vi "Handle Last Ack Core.vi"(4 "error in (no error)":errorcluster, 6 "Last Ack":refnum<class "Last Ack.lvclass">, 7 "MultiplexedConnectionHandler in":refnum<class "MultiplexedConnectionHandler.lvclass">) -> (0 "error out":errorcluster, 3 "MultiplexedConnectionHandler out":refnum<class "MultiplexedConnectionHandler.lvclass">)   [LabVIEW 2019, in "MultiplexedConnectionHandler.lvlib" / "MultiplexedConnectionHandler.lvclass"]
doc: "(<B>Filename</B>: Actor Framework.lvlib:Actor.lvclass:Handle Last Ack Core.vi)\n\nDefines how the caller actor responds to the Last Ack message from a nested actor. The Last Ack message is the final message a nested actor sends to its caller before it shuts down. The message contains information about the final state of the nested actor.\n\nBy default, this method does nothing except return any error the nested actor sent. A descendant class may override this method to define behavior."
uses:
  <vilib>/gpm_packages/@cs/Network-interface/Source/MultiplexedConnectionHandler/MultiplexedConnectionHandler/MultiplexedConnectionHandler.lvclass
  <vilib>/ActorFramework/LastAck/Last Ack.lvclass
  C:/Program Files/National Instruments/LabVIEW 2019/vi.lib/gpm_packages/@cs/Network-interface/Source/PersistantConnectionHandler/PersistantConnectionHandler/PersistantConnectionHandler.lvclass
  C:/Program Files/National Instruments/LabVIEW 2019/vi.lib/gpm_packages/@cs/Network-interface/Source/Logged Actor/LoggedActor.lvclass
  <vilib>/gpm_packages/@cs/Network-interface/Source/ConnectionManager/ConnectionManager/ConnectionManager.lvclass
  <vilib>/gpm_packages/@cs/event-logger/Source/Composed Log/Types/Log Level.ctl
  <vilib>/ActorFramework/LastAck/Last Ack.lvclass/Last Ack.ctl
  <vilib>/gpm_packages/@cs/Network-interface/Source/PersistantConnectionHandler/PersistantConnectionHandler/PersistantConnectionHandler.lvclass/PersistantConnectionHandler.ctl
  <vilib>/gpm_packages/@cs/Network-interface/Source/MultiplexedConnectionHandler/MultiplexedConnectionHandler/MultiplexedConnectionHandler.lvclass/MultiplexedConnectionHandler.ctl
  <vilib>/gpm_packages/@cs/Network-interface/Source/ConnectionManager/ConnectionManager/ConnectionManager.lvclass/ConnectionManager.ctl
  <vilib>/ActorFramework/Message Enqueuer/Message Enqueuer.lvclass
  <vilib>/gpm_packages/@cs/Network-interface/Source/Connection Reference/Connection Reference/Connection Reference.lvclass
  <vilib>/gpm_packages/@cs/Network-interface/Source/Logged Actor/LoggedActor.lvclass/LoggedActor.ctl
  <vilib>/gpm_packages/@cs/event-logger/Source/Composed Log/LoggerReference/LoggerReference.lvclass/LoggerReference.ctl
  <vilib>/gpm_packages/@cs/event-logger/Source/Composed Log/LoggerReference/Log Event.vi
  <vilib>/gpm_packages/@cs/event-logger/Source/Composed Log/LoggerReference/Log.vi
  <vilib>/gpm_packages/@cs/event-logger/Source/Composed Log/LoggerReference/Get Valid Event Time.vi
  <vilib>/gpm_packages/@cs/event-logger/Source/Composed Log/LoggerReference/Remove Stale Logs.vi
  <vilib>/gpm_packages/@cs/Network-interface/Source/MessagingInterfaces/IConnectionStateChangeCallback/IConnectionStateChangeCallback.lvclass
  <vilib>/gpm_packages/@cs/Network-interface/Source/Logged Actor/LoggedActor.lvclass
  <vilib>/gpm_packages/@cs/event-logger/Source/Composed Log/Composed Log.lvlib
  <vilib>/gpm_packages/@cs/Network-interface/Source/PersistantConnectionHandler/PersistantConnectionHandler/PersistantConnectionHandler.lvclass
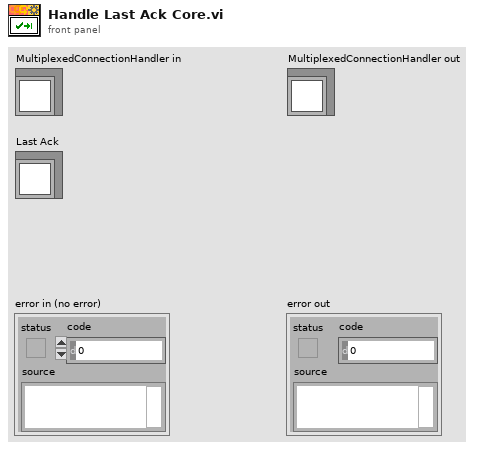
[diagram p1: front panel]
types:
  T1 = typedef "Composed Log.lvlib/Log Level.ctl" = enum16{"Debug", "Info", "Warning", "Error", "Critical"}
  T2 = cluster{"Connection Manager Queue":refnum<class "Message Enqueuer.lvclass">, "Connection Reference":refnum<data-value>}
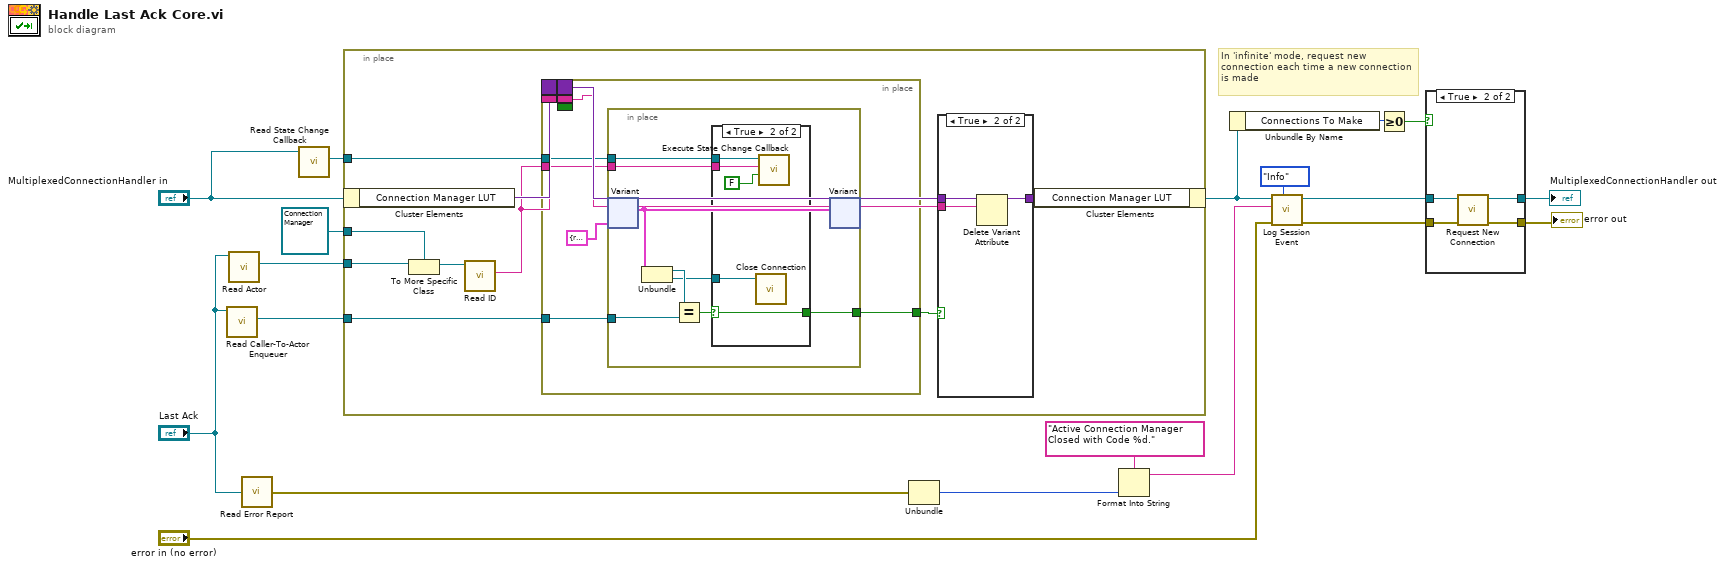
[diagram p0: block diagram]
diagram:
  # "In 'infinite' mode, request new connection each time a new connection is made"
  n1 = call <vilib>:"Read Caller-To-Actor Enqueuer.vi"("Last Ack"="Last Ack") -> ("Caller-to-Actor Enqueuer"=w15:refnum<class "Message Enqueuer.lvclass">)  [unwired: 10 in]
  n2 = call <vilib>:"Read Actor.vi"("Last Ack"="Last Ack") -> ("Actor"=w11:refnum<class "Actor.lvclass">)  [unwired: 10 in]
  n3 = call <vilib>:"Read Error Report.vi"("Last Ack"="Last Ack") -> ("error report"=w19:errorcluster)
  n4 = call <vilib>:"Read State Change Callback.vi"("PersistantConnectionHandler in"="MultiplexedConnectionHandler in") -> ("State Change Callback"=w1:refnum<class "IConnectionStateChangeCallback.lvclass">)  [unwired: 9 in, 1 out]
  n5 = in-place {
    in-place-border: w15 -> [w29]
    in-place-border: refnum<class "ConnectionManager.lvclass"> refnum ("ConnectionManager.lvlib:ConnectionManager.lvclass") -> [w24]
    in-place-border: w11 -> [w23]
    in-place-border: w1 -> [w21]
    n6 = in-place-cluster #1("MultiplexedConnectionHandler in") -> ("Connection Manager LUT"=w30:variant)
    n7 = To More Specific Class(target class=w24, reference=w23) -> (specific class reference=w22:refnum<class "ConnectionManager.lvclass">)  [unwired: 1 in, 1 out]
    n8 = call <vilib>:"Read ID.vi"("ConnectionManager in"=w22) -> ("ID"=w20:string)  [unwired: 8 in, 2 out]
    n9 = in-place {
      border: w30 -> [_]
      border: w20 -> [_]
      border: [_] -> w28
      border: [_] -> w25
      border: _ -> [_]
      in-place-border: w29 -> [w38]
      in-place-border: [w37] -> w27
      in-place-border: w21 -> [w36]
      in-place-border: w20 -> [w35]
      n10 = in-place {
        in-place-border: w38 -> [w48]
        in-place-border: [w44] -> w37
        in-place-border: w36 -> [w43]
        in-place-border: w35 -> [w42]
        n11 = in-place-variant #2(w41, T2 {"Connection Manager Queue"=refnum, "Connection Reference"=refnum}) -> (w49:T2)  [unwired: 1 out]
        n12 = Unbundle(w49) -> ("Connection Manager Queue"=w47:refnum<class "Message Enqueuer.lvclass">, "Connection Reference"=w45:refnum<data-value>)
        n13 = Equal?(x=w47, y=w48) -> (x = y?=w46:bool)
        n14 = case shown="True" w46 {
          selector: w46 -> [w50 w54]
          tunnel: w45 -> [_ w55]
          tunnel: [w50 w54] -> w44
          tunnel: w43 -> [_ w53]
          tunnel: w42 -> [_ w52]
          frame False {
          }
          frame True {
            n15 = call <vilib>:"Close Connection.vi"("Connection Reference In"=w55) -> ()  [unwired: 10 in, 1 out]
            n16 = call-dynamic "Execute State Change Callback.vi"("Connection State"=FALSE, "Connection ID"=w52, "IConnectionStateChangeCallback in"=w53) -> ()  [unwired: 8 in, 1 out]
          }
        }
        n17 = in-place-variant #2(w49) -> (w40:variant)  [unwired: 1 out]
      }
    }
    n18 = case shown="True" w27 {
      tunnel: w28 -> [w31 w34]
      tunnel: [w31 w33] -> w26
      tunnel: w25 -> [_ w32]
      frame False {
      }
      frame True {
        n19 = Delete Variant Attribute(6:w32, 7:w34) -> (3:w33:variant)  [unwired: 1 in, 2 out]
      }
    }
    n20 = in-place-cluster #1("Connection Manager LUT"=w26) -> (w5:refnum<class "MultiplexedConnectionHandler.lvclass">)
  }
  n21 = Unbundle(w19) -> ("code"=w18:i32)  [unwired: 2 out]
  n22 = Format Into String(format string="Active Connection Manager Closed with Code %d.", w18) -> (resulting string=w14:string)  [unwired: 2 in, 1 out]
  n23 = Unbundle By Name(w5) -> ("Connections To Make"=w4:i32)
  n24 = call <vilib>:"Log Session Event.vi"("Event Level"=Log_Level."Info", "error in (no error)"="error in (no error)", "Event Data"=w14, "SessionActor in"=w5) -> ("error out"=w8:errorcluster, "SessionActor out"=w9:refnum<class "MultiplexedConnectionHandler.lvclass">)  [unwired: 6 in]
  n25 = Greater Or Equal To 0?(x=w4) -> (x >= 0?=w3:bool)
  n26 = case shown="True" w3 {
    tunnel: w9 -> [w57 w61]
    tunnel: w8 -> [w56 w60]
    tunnel: [w56 w59] -> w7
    tunnel: [w57 w58] -> w6
    frame False {
    }
    frame True {
      n27 = call <vilib>:"Request New Connection.vi"("error in (no error)"=w60, "PersistantConnectionHandler in"=w61) -> ("error out"=w59:errorcluster, "PersistantConnectionHandler out"=w58:refnum<class "MultiplexedConnectionHandler.lvclass">)  [unwired: 8 in]
    }
  }
  "MultiplexedConnectionHandler out" <- w6
  "error out" <- w7
